vi "Blob Detection.vi"(7 "Ring Light Color":T2={"Hue"={119.53551591960586, 182.50767725024022}, "Sat"={103.21428571428572, 255.0}, "Val"={133.57142857142858, 255.0}} {"Hue" scale=0.0..255.0 scale format="%#_3g"}, 10 "Image":T1) -> (0 "HSL Image":T1, 3 "Acceptable Blobs":T3(array[cluster]), 4 "Image 2":T1)   [LabVIEW 2014]
uses:
  <vilib>/vision/Image Controls.llb/IMAQ Image.ctl
  <vilib>/vision/NI_Vision_Development_Module.lvlib
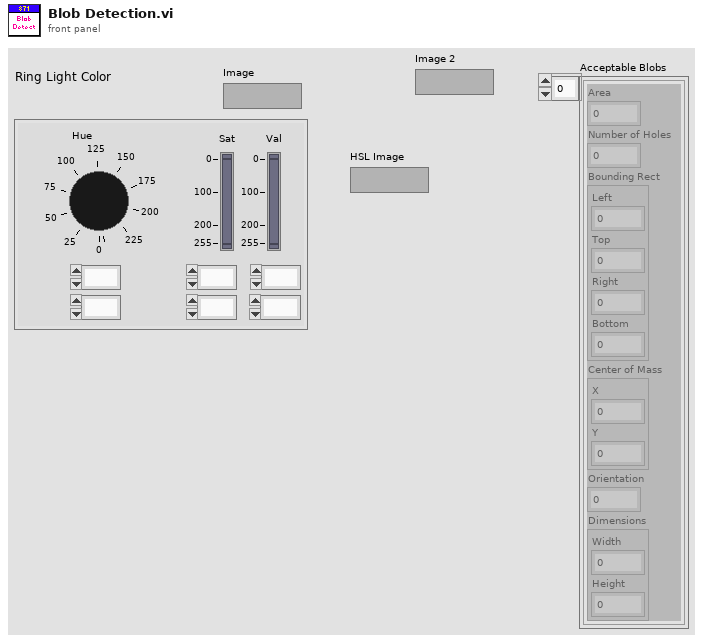
[diagram p1: front panel]
types:
  T1 = typedef "IMAQ Image.ctl" = refnum<image>
  T2 = cluster{"Hue":cluster{dbl, dbl}, "Sat":cluster{dbl, dbl}, "Val":cluster{dbl, dbl}}
  T3 = cluster{"Area":dbl, "Number of Holes":dbl, "Bounding Rect":cluster{"Left":dbl, "Top":dbl, "Right":dbl, "Bottom":dbl}, "Center of Mass":cluster{"X":dbl, "Y":dbl}, "Orientation":dbl, "Dimensions":cluster{"Width":dbl, "Height":dbl}}[]
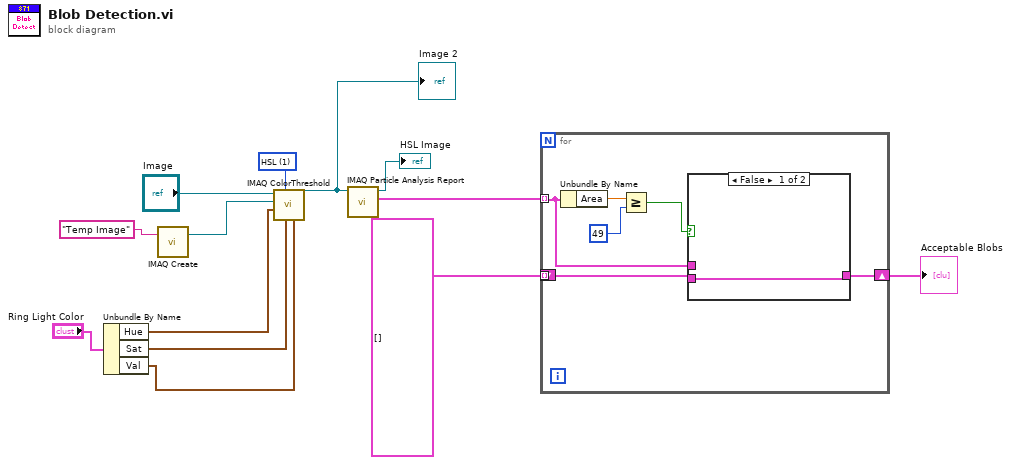
[diagram p0: block diagram]
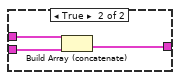
[diagram p2: hidden frame]
diagram:
  w13 = u16 1 items=["RGB", "HSL", "HSV", "HSI"] ("Color Mode")
  n1 = Unbundle By Name("Ring Light Color") -> ("Hue"=w8:cluster{dbl, dbl}, "Sat"=w7:cluster{dbl, dbl}, "Val"=w6:cluster{dbl, dbl})
  n2 = call "IMAQ Create"("Image Name"="Temp Image") -> ("New Image"=w3:T1)  [unwired: 4 in, 1 out]
  n3 = call "IMAQ ColorThreshold"("Blue or Luma or Val or Inten Range"=w6, "Green or Sat Range"=w7, "Color Mode"=w13, "Red or Hue Range"=w8, "Image Dst"=w3, "Image Src"="Image") -> ("Image Dst Out"=w2:T1)  [unwired: 4 in, 1 out]
  "Image 2" <- w2
  n4 = call "IMAQ Particle Analysis Report"("Image"=w2) -> ("Particle Reports (Pixels)"=w12:T3, "Image Out (duplicate)"=→"HSL Image":T1)  [unwired: 5 in, 4 out]
  n5 = for {
    tunnel: w12 -> [w16] mode=indexing
    shift-right: [w15] -> w11
    shift-left: T3 [] ("Acceptable Blobs 2") -> [w14]
    tunnel: [w14] -> _ mode=indexing
    n6 = Unbundle By Name(w16) -> ("Area"=w19:dbl)
    n7 = Greater Or Equal?(x=w19, y=49) -> (x >= y?=w17:bool)
    n8 = case shown="False" w17 {
      tunnel: w16 -> [_ w22]
      tunnel: [w20 w23] -> w15
      tunnel: w14 -> [w20 w21]
      frame False {
      }
      frame True {
        n9 = Build Array (concatenate)(w22, w21) -> (w23:T3)
      }
    }
  }
  "Acceptable Blobs" <- w11
